vi "(FPGA)_PIDXYZ_laserPID)_COMtemp.vi"() -> ()   [LabVIEW 2018]
doc: "This VI will read single point values from 4 channels of a R Series board at a specified rate."
uses:
  <vilib>/rvi/Emulation/niFpgaGetClockAttributes.vi
  <vilib>/rvi/Emulation/niFpgaSctlEmulationGetInTimedLoop.vi
  <vilib>/rvi/Emulation/niFpgaEmulationReportErrorSimple.vi
  <vilib>/rvi/Emulation/niFpgaProcessEmulError.vi
  <vilib>/rvi/eio/common/nirviEmuTemplateMethod_errors.vi
  <vilib>/rvi/Emulation/niFpgaCriticalErrorInLSC.vi
  <vilib>/rvi/Memory/Memory_Emulation/nirvimemoryFastEmulation.vi
  <vilib>/rvi/Memory/Memory_Emulation/nirvimemoryEmulation.vi
  <vilib>/rvi/Emulation/niFpgaEmulationIsFPGAContextNoSignature.vi
  <vilib>/rvi/DataTransferAndStorage/Container/Common/niFpgaContainerGetUniqueNameForEmu.vi
  <vilib>/rvi/errors/nirviReportUnexpectedCaseInternalError (U32).vi
  <vilib>/rvi/Memory/Memory_Emulation/niFpgaMemoryEmulationCacheClearOnFirstRun.vi
  <vilib>/rvi/Memory/Memory_Emulation/nirvimemoryEmulationManagerCache_MakeExclusive.vi
  <vilib>/rvi/Memory/Memory_Emulation/niFpgaMemoryEmulationValidateCache.vi
  <vilib>/rvi/Memory/Memory_Emulation/nirvimemoryEmulationManagerCache_InsertValue.vi
  <vilib>/Utility/error.llb/Clear Errors.vi
  <vilib>/rvi/Memory/Memory_Emulation/nirvimemoryEmulationManagerCache_ReleaseExclusive.vi
  <vilib>/rvi/Memory/Memory_Emulation/nirvimemoryEmulationManagerCache_GetValue.vi
  <vilib>/rvi/Memory/Memory_Emulation/nirvimemoryEmulationManagerCache_SetValue.vi
  <vilib>/rvi/Emulation/niFpgaSctlEmulationResourceMgr.vi
  <vilib>/eio/EIONode/EIONode.xnode
  <vilib>/rvi/DataTransferAndStorage/Container/XNode/niFpgaContainer.xnode
  <vilib>/rvi/FXPMathLib/FxpInterpret/XNode/nifxpmath_Interpret.xnode
panel:
  in  "Big Number":sgl
  in  "Amplitude_sine_EOM":sgl
  in  "eom sine frequency (periods/tick)":fxp<+,32,0>=0.0002500000409781933
  in  "pz?":bool
  out "pg Z mod":fxp<+/-,24,12>
  in  "pg Z":fxp<+/-,24,12>
  in  "amplitude":i16=8192
  in  "offset":i16=8192
  out "Trigger for COM out":i16 caption="square wave out"
  out "dgz mod":fxp<+/-,24,12>
  in  "activate COMz":bool
  in  "dg Z":fxp<+/-,24,12>
  in  "activate COMy":bool
  out "dgy mod":fxp<+/-,24,12>
  in  "dg Y":fxp<+/-,24,12>
  out "dgx mod":fxp<+/-,24,12>
  in  "activate COMx":bool
  in  "dg X":fxp<+/-,24,12>
  in  "duty cycle (periods)":fxp<+,32,0>=0.5
  in  "frequency (periods/tick)":fxp<+,32,0>=0.00390625
  in  "final filter coeff X before":i32[](array[numeric])=[-955995012, 2025731616, 1001305, -1023351008, 2092954700, 1034533]
  in  "final filter coeff X":i32[](array[numeric])=[-955995012, 2025731616, 1001305, -1023351008, 2092954700, 1034533]
  in  "final filter coeff Y before":i32[](array[numeric])=[-955995012, 2025731616, 1001305, -1023351008, 2092954700, 1034533]
  in  "final filter coeff Y":i32[](array[numeric])=[-955995012, 2025731616, 1001305, -1023351008, 2092954700, 1034533]
  in  "final filter coeff Z":i32[](array[numeric])=[-955995012, 2025731616, 1001305, -1023351008, 2092954700, 1034533]
  in  "final filter coeff Z before":i32[](array[numeric])=[-955995012, 2025731616, 1001305, -1023351008, 2092954700, 1034533]
  in  "LP Coeff Z before":i32[](array[numeric])=[1008310688, 32715568]
  in  "LP Coeff Z":i32[](array[numeric])=[1008310688, 32715568]
  in  "LP Coeff X":i32[](array[numeric])=[1008310688, 32715568]
  in  "LP Coeff X before":i32[](array[numeric])=[1008310688, 32715568]
  in  "LP Coeff Y before":i32[](array[numeric])=[1008310688, 32715568]
  in  "LP Coeff Y":i32[](array[numeric])=[1008310688, 32715568]
  in  "Upper lim Z before":fxp<+/-,16,16>
  in  "Lower lim Z before":fxp<+/-,16,16>
  in  "Upper lim Y before":fxp<+/-,16,16>
  in  "Lower lim Y before":fxp<+/-,16,16>
  in  "Upper lim X before":fxp<+/-,16,16>
  in  "Lower lim X before":fxp<+/-,16,16>
  in  "HP coeff band X before":i32[](array[numeric])=[-850883994, 1909449570, 958518847, -975456236, 2033039520, 1020559395]
  in  "LP Coeff band X before":i32[](array[numeric])=[-955995012, 2025731616, 1001305, -1023351008, 2092954700, 1034533]
  in  "LP Coeff band X":i32[](array[numeric])=[-955995012, 2025731616, 1001305, -1023351008, 2092954700, 1034533]
  in  "HP Coeff band X":i32[](array[numeric])=[-850883994, 1909449570, 958518847, -975456236, 2033039520, 1020559395]
  in  "dg band X before":fxp<+/-,24,12>
  in  "dg band X":fxp<+/-,24,12>
  in  "HP Coeff X before":i32[](array[numeric])=[946630756, 1010186290]
  in  "HP Coeff X":i32[](array[numeric])=[946630756, 1010186290]
  in  "Use X PID before":bool
  out "AI X before chamber plot":i16
  in  "X before Setpoint":i16
  out "tot_fb X plot":i16
  out "fb X before chamber plot":i16
  in  "DC offset X":i16
  in  "pg X before":fxp<+/-,24,12>
  in  "ig X before":fxp<+/-,24,-4>
  in  "dg X before":fxp<+/-,24,12>
  out "fb X plot":i16
  in  "ig X":fxp<+/-,24,-4>
  in  "Lower lim X":fxp<+/-,16,16>
  in  "Upper lim X":fxp<+/-,16,16>
  in  "pg X":fxp<+/-,24,12>
  out "AI X plot":i16
  in  "X Setpoint":i16
  in  "HP coeff band Y before":i32[](array[numeric])=[-850883994, 1909449570, 958518847, -975456236, 2033039520, 1020559395]
  in  "LP Coeff band Y before":i32[](array[numeric])=[-955995012, 2025731616, 1001305, -1023351008, 2092954700, 1034533]
  in  "LP Coeff band Y":i32[](array[numeric])=[-955995012, 2025731616, 1001305, -1023351008, 2092954700, 1034533]
  in  "HP Coeff band Y":i32[](array[numeric])=[-850883994, 1909449570, 958518847, -975456236, 2033039520, 1020559395]
  in  "dg band Y before":fxp<+/-,24,12>
  in  "dg band Y":fxp<+/-,24,12>
  in  "HP Coeff Y before":i32[](array[numeric])=[946630756, 1010186290]
  in  "HP Coeff Y":i32[](array[numeric])=[946630756, 1010186290]
  in  "Use Y PID before":bool
  out "AI Y before chamber plot":i16
  in  "Y before Setpoint":i16
  out "tot_fb Y plot":i16
  out "fb Y before chamber plot":i16
  in  "DC offset Y":i16
  in  "pg Y before":fxp<+/-,24,12>
  in  "ig Y before":fxp<+/-,24,-4>
  in  "dg Y before":fxp<+/-,24,12>
  out "fb Y plot":i16
  in  "ig Y":fxp<+/-,24,-4>
  in  "Lower lim Y":fxp<+/-,16,16>
  in  "Upper lim Y":fxp<+/-,16,16>
  in  "pg Y":fxp<+/-,24,12>
  out "AI Y plot":i16
  in  "Y Setpoint":i16
  in  "EOM_offset":i16
  in  "EOM_seed":u32=4294967295 caption="seed"
  in  "EOM reset":bool caption="reset"
  in  "EOM_threshold":i16
  in  "EOM_amplitude":i16
  in  "HP coeff band Z before":i32[](array[numeric])=[-850883994, 1909449570, 958518847, -975456236, 2033039520, 1020559395]
  in  "LP Coeff band Z before":i32[](array[numeric])=[-955995012, 2025731616, 1001305, -1023351008, 2092954700, 1034533]
  in  "LP Coeff band Z":i32[](array[numeric])=[-955995012, 2025731616, 1001305, -1023351008, 2092954700, 1034533]
  in  "HP Coeff band Z":i32[](array[numeric])=[-850883994, 1909449570, 958518847, -975456236, 2033039520, 1020559395]
  in  "dg band Z before":fxp<+/-,24,12>
  in  "dg band Z":fxp<+/-,24,12>
  in  "data_buffer3":i16
  in  "Arb gain (ch2)":fxp<+/-,24,12>=0.5 caption="RMS"
  in  "HP Coeff Z before":i32[](array[numeric])=[946630756, 1010186290]
  in  "HP Coeff Z":i32[](array[numeric])=[946630756, 1010186290]
  in  "Use Z PID before":bool
  out "AI Z before chamber plot":i16
  in  "Z before Setpoint":i16
  out "tot_fb Z plot":i16
  out "fb Z before chamber plot":i16
  in  "DC offset Z":i16
  in  "pg Z before":fxp<+/-,24,12>
  in  "ig Z before":fxp<+/-,24,-4>
  in  "dg Z before":fxp<+/-,24,12>
  out "fb Z plot":i16
  in  "ig Z":fxp<+/-,24,-4>
  out "written_address":u32
  in  "ready_to_write":bool
  in  "Arb steps per cycle":u16
  in  "data_buffer2":i16
  in  "data_buffer_1":i16
  in  "write_address":u16
  in  "Arb gain (ch1)":fxp<+/-,24,12>=0.5 caption="RMS"
  in  "Arb gain (ch0)":fxp<+/-,24,12>=0.5 caption="RMS"
  in  "Lower lim Z":fxp<+/-,16,16>
  in  "Upper lim Z":fxp<+/-,16,16>
  out "AI Z plot":i16
  in  "Z Setpoint":i16
  in  "Count(uSec)":u32
  out "FPGA Error Out":errorcluster
  in  "Stop":bool
  # "test"
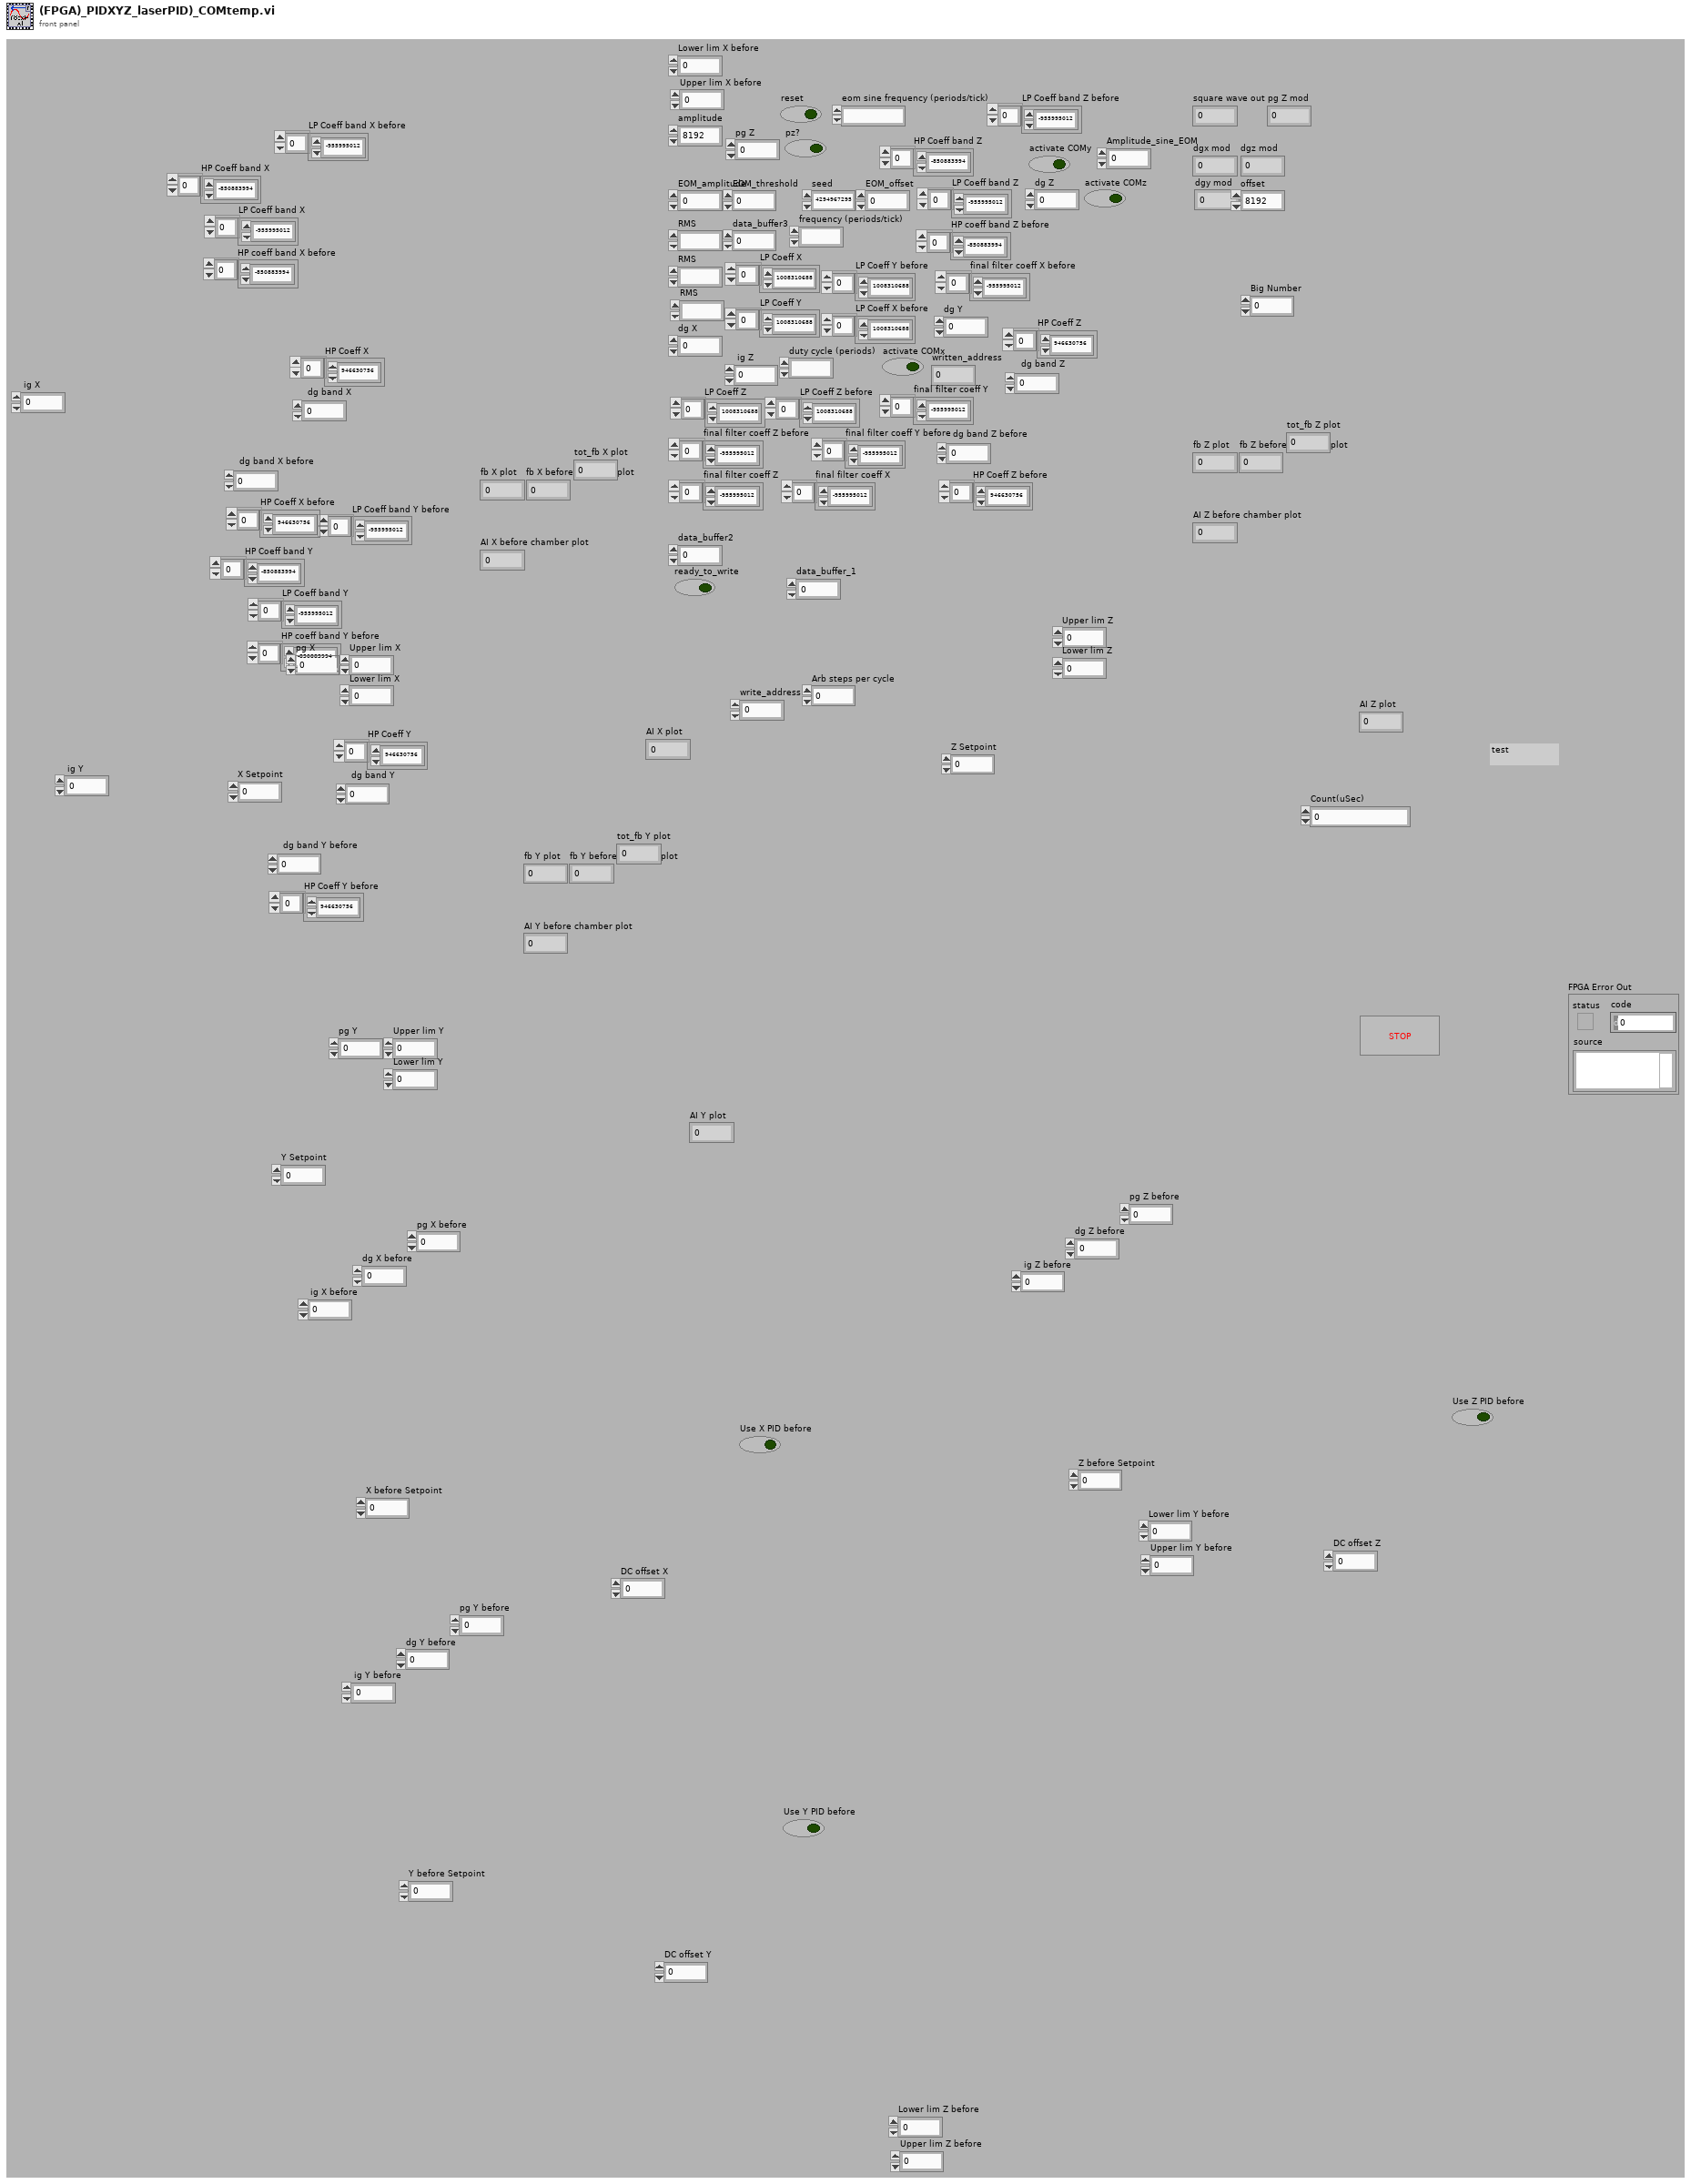
[diagram p1: front panel]
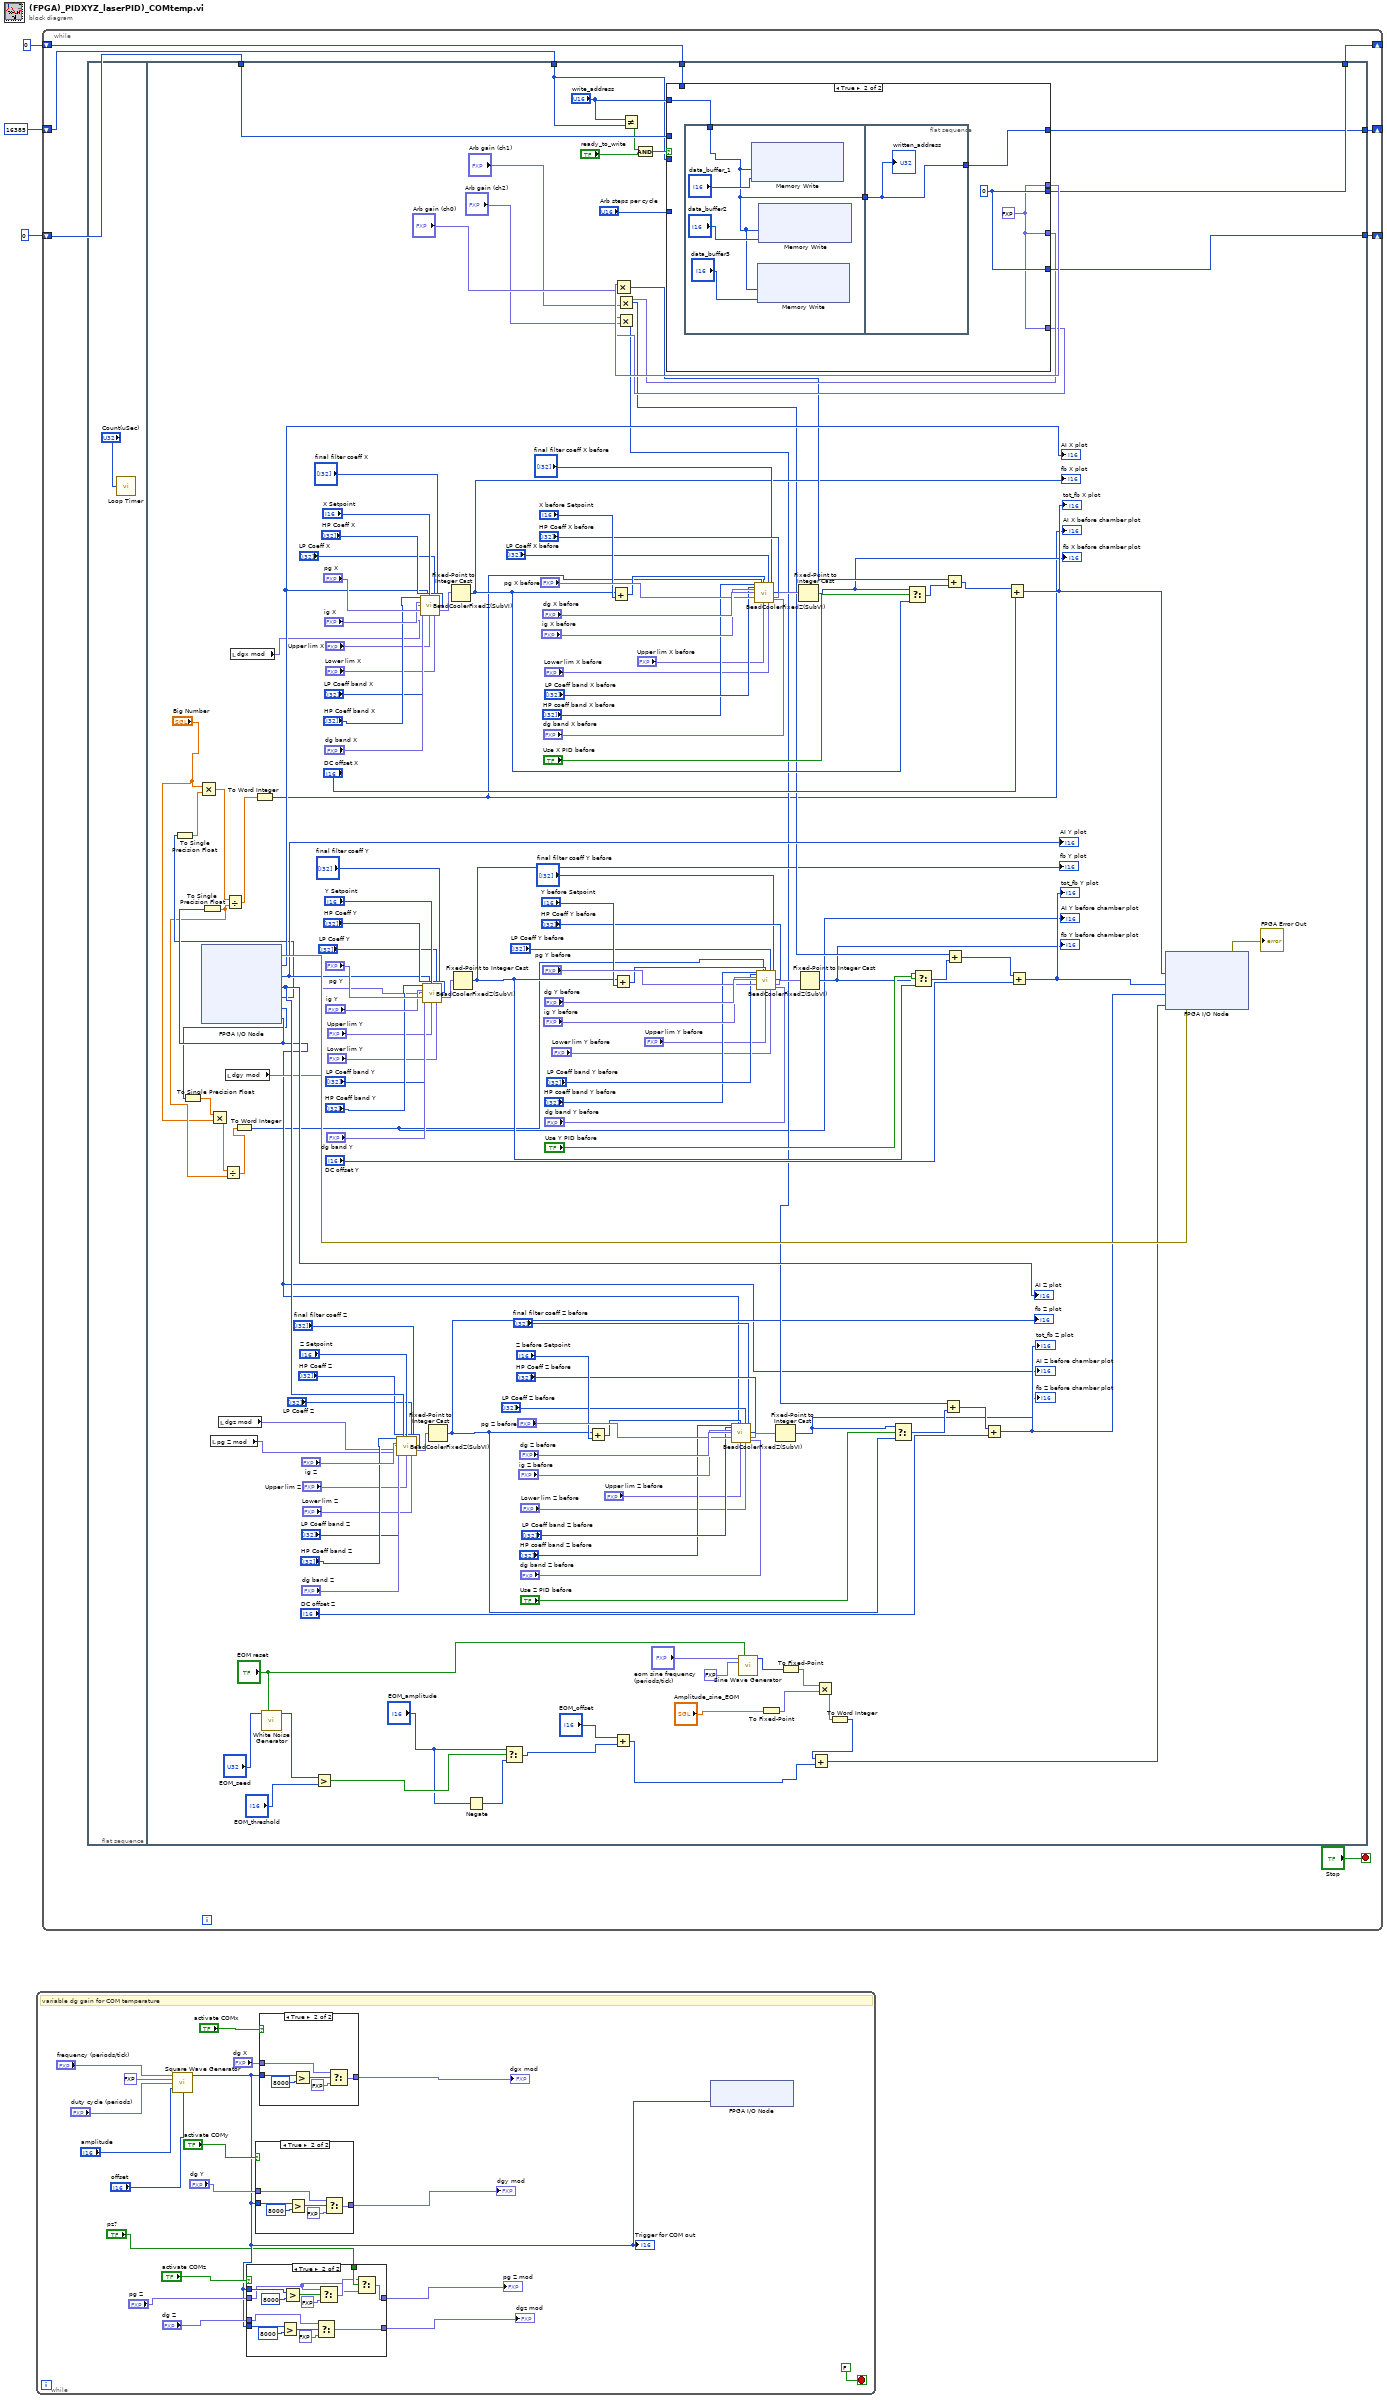
[diagram p0: block diagram]
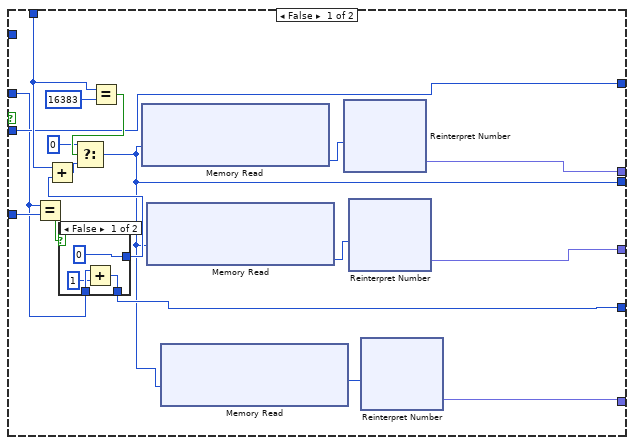
[diagram p5: hidden frame]
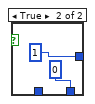
[diagram p6: hidden frame]
diagram:
  n1 = while {
    stop <- FALSE stop-if-true
    # "variable dg gain for COM temperature"
    n2 = call "Square Wave Generator"("frequency (periods/tick)"="frequency (periods/tick)", "phase offset (periods)"=fxp<+,32,0> 0.0, "duty cycle (periods)"="duty cycle (periods)", "amplitude"="amplitude", "offset"="offset") -> ("square wave out"=w5:i16)  [unwired: 10 in]
    "Trigger for COM out" <- w5
    n3 = case shown="True" "activate COMz" {
      tunnel: [w24 w35] -> w8
      tunnel: w5 -> [_ w38]
      tunnel: "dg Z" -> [w24 w33]
      tunnel: "pg Z" -> [w23 w25]
      tunnel: [w23 w26] -> w6
      tunnel: w5 -> [_ w29]
      tunnel: "pz?" -> [_ w28]
      frame False {
      }
      frame True {
        n4 = Greater?(x=w38, y=i16 8000) -> (0:w36:bool)
        n5 = Greater?(x=w29, y=i16 8000) -> (0:w31:bool)
        n6 = Select(t=w33, s=w36, f=fxp<+/-,24,12> 0.0 ("y")) -> (s? t:f=w35:fxp<+/-,24,12>)
        n7 = Select(t=w25, s=w31, f=fxp<+/-,24,12> 0.0 ("y")) -> (s? t:f=w27:fxp<+/-,24,12>)
        n8 = Select(t=w27, s=w28, f=w25) -> (s? t:f=w26:fxp<+/-,24,12>)
      }
    }
    "dgz mod" <- w8
    "pg Z mod" <- w6
    n9 = case shown="True" "activate COMy" {
      tunnel: "dg Y" -> [w39 w41]
      tunnel: [w39 w42] -> w12
      tunnel: w5 -> [_ w45]
      frame False {
      }
      frame True {
        n10 = Greater?(x=w45, y=i16 8000) -> (0:w43:bool)
        n11 = Select(t=w41, s=w43, f=fxp<+/-,24,12> 0.0 ("y")) -> (s? t:f=w42:fxp<+/-,24,12>)
      }
    }
    "dgy mod" <- w12
    n12 = case shown="True" "activate COMx" {
      tunnel: "dg X" -> [w46 w48]
      tunnel: [w46 w49] -> w14
      tunnel: w5 -> [_ w52]
      frame False {
      }
      frame True {
        n13 = Greater?(x=w52, y=i16 8000) -> (0:w50:bool)
        n14 = Select(t=w48, s=w50, f=fxp<+/-,24,12> 0.0 ("y")) -> (s? t:f=w49:fxp<+/-,24,12>)
      }
    }
    "dgx mod" <- w14
    n15 = xnode "FPGA I/O Node"("Connector0/AO7"=w5) -> ()  [unwired: 2 in, 2 out]
  }
  n16 = while {
    shift-right: [w58] -> _
    shift-left: u16 0 ("t") -> [w57]
    shift-right: [w56] -> _
    shift-left: u16 0 ("t") -> [w53]
    shift-right: [w55] -> _
    shift-left: u32 16385 ("write_address") -> [w54]
    stop <- "Stop" stop-if-true
    n17 = flat-sequence {
      tunnel: [w214] -> w58
      tunnel: w57 -> [w213]
      tunnel: [w211] -> w56
      tunnel: w53 -> [w210]
      tunnel: [w209] -> w55
      tunnel: w54 -> [w202]
      frame #0 {
        n18 = call "Loop Timer"("Count(uSec)"="Count(uSec)") -> ()  [unwired: 1 out]
      }
      frame #1 {
        n19 = xnode "FPGA I/O Node"() -> ("error out"=w219:errorcluster, "Connector0/AI0"=w123:i16, "Connector0/AI1"=w147:i16, "Connector0/AI2"=w200:i16, "Connector0/AI3"=w68:i16, "Connector0/AI4"=w67:i16, "Connector0/AI5"=w72:i16)  [unwired: 7 in, 6 out]
        "AI Z plot" <- w200
        "AI Z before chamber plot" <- w72
        "AI Y plot" <- w147
        "AI X plot" <- w123
        n20 = To Single Precision Float(number=w68) -> (single precision float=w71:sgl)
        n21 = To Single Precision Float(number=w67) -> (single precision float=w66:sgl)
        n22 = Multiply(x="Big Number", y=w71) -> (x*y=w70:sgl)
        n23 = To Single Precision Float(number=w72) -> (single precision float=w64:sgl)
        n24 = Multiply(x=w66, y="Big Number") -> (x*y=w65:sgl)
        n25 = local read "pg Z mod"() -> (w85:fxp<+/-,24,12>)
        n26 = local read "dgz mod"() -> (w86:fxp<+/-,24,12>)
        n27 = Divide(x=w65, y=w64) -> (x/y=w63:sgl)
        n28 = Divide(x=w70, y=w64) -> (x/y=w69:sgl)
        n29 = local read "dgy mod"() -> (w87:fxp<+/-,24,12>)
        n30 = local read "dgx mod"() -> (w88:fxp<+/-,24,12>)
        n31 = To Word Integer(number=w63) -> (16bit integer=w62:i16)
        "AI Y before chamber plot" <- w62
        n32 = To Word Integer(number=w69) -> (16bit integer=w73:i16)
        "AI X before chamber plot" <- w73
        n33 = call "White Noise Generator"("seed"="EOM_seed", "reset"="EOM reset") -> ("white noise out"=w179:i16)  [unwired: 13 in]
        n34 = Greater?(x=w179, y="EOM_threshold") -> (0:w177:bool)
        n35 = call "BeadCoolerFixedZ(SubVI).vi"("hp coeff band"="HP Coeff band Z", "lp coeff band"="LP Coeff band Z", "ig"="ig Z", "dg"=w86, "pg"=w85, "dg band"="dg band Z", "AI0"=w200, "Dc Pos"="Z Setpoint", "Upper lim"="Upper lim Z", "lp coeff"="LP Coeff Z", "Lower lim"="Lower lim Z", "final filter coeff"="final filter coeff Z", "hp coeff"="HP Coeff Z") -> ("Output"=w189:fxp<+/-,16,16>)  [unwired: 14 in]
        n36 = call "BeadCoolerFixedZ(SubVI).vi"("hp coeff band"="HP Coeff band X", "lp coeff band"="LP Coeff band X", "ig"="ig X", "dg"=w88, "pg"="pg X", "dg band"="dg band X", "AI0"=w123, "Dc Pos"="X Setpoint", "Upper lim"="Upper lim X", "lp coeff"="LP Coeff X", "Lower lim"="Lower lim X", "final filter coeff"="final filter coeff X", "hp coeff"="HP Coeff X") -> ("Output"=w133:fxp<+/-,16,16>)  [unwired: 14 in]
        n37 = call "BeadCoolerFixedZ(SubVI).vi"("hp coeff band"="HP Coeff band Y", "lp coeff band"="LP Coeff band Y", "ig"="ig Y", "dg"=w87, "pg"="pg Y", "dg band"="dg band Y", "AI0"=w147, "Dc Pos"="Y Setpoint", "Upper lim"="Upper lim Y", "lp coeff"="LP Coeff Y", "Lower lim"="Lower lim Y", "final filter coeff"="final filter coeff Y", "hp coeff"="HP Coeff Y") -> ("Output"=w157:fxp<+/-,16,16>)  [unwired: 14 in]
        n38 = Fixed-Point to Integer Cast(1:w189) -> (0:w98:i16)
        "fb Z plot" <- w98
        n39 = Fixed-Point to Integer Cast(1:w133) -> (0:w102:i16)
        "fb X plot" <- w102
        n40 = Fixed-Point to Integer Cast(1:w157) -> (0:w100:i16)
        "fb Y plot" <- w100
        n41 = Negate(x="EOM_amplitude") -> (-x=w175:i16)
        n42 = Select(t="EOM_amplitude", s=w177, f=w175) -> (s? t:f=w173:i16)
        n43 = Add(x=w98, y="Z before Setpoint") -> (x+y=w188:i16)
        n44 = Add(x=w102, y="X before Setpoint") -> (x+y=w132:i16)
        n45 = Add(x=w100, y="Y before Setpoint") -> (x+y=w156:i16)
        n46 = Add(x="EOM_offset", y=w173) -> (x+y=w76:i16)
        n47 = Not Equal?(x="write_address", y=w202) -> (x != y?=w206:bool)
        n48 = And(x=w206, y="ready_to_write") -> (x .and. y?=w207:bool)
        n49 = case shown="True" w207 {
          tunnel: [w236 w244] -> w216
          tunnel: [w221 w248] -> w214
          tunnel: w213 -> [w229 _]
          tunnel: [w230 w244] -> w204
          tunnel: "Arb steps per cycle" -> [w228 _]
          tunnel: [w223 w248] -> w211
          tunnel: w210 -> [w224 _]
          tunnel: [w227 w246] -> w209
          tunnel: w202 -> [w227 _]
          tunnel: "write_address" -> [_ w245]
          tunnel: [w220 w244] -> w186
          frame False {
            n50 = Equal?(x=w224, y=w228) -> (x = y?=w226:bool)
            n51 = case shown="False" w226 {
              tunnel: [u16 0 ("y") u16 1 ("y")] -> w225
              tunnel: w224 -> [w240 _]
              tunnel: [w238 u16 0] -> w223
              frame False {
                n52 = Add(x=w240, y=u16 1) -> (x+y=w238:u16)
              }
              frame True {
              }
            }
            n53 = Add(x=w229, y=w225) -> (x+y=w232:u16)
            n54 = Equal?(x=w229, y=u16 16383) -> (x = y?=w234:bool)
            n55 = Select(t=u16 0, s=w234, f=w232) -> (s? t:f=w221:u16)
            n56 = xnode ("Memory Read")("Address"=w221) -> ("Data"=w237:i16)  [unwired: 1 in, 1 out]
            n57 = xnode ("Memory Read")("Address"=w221) -> ("Data"=w231:i16)  [unwired: 1 in, 1 out]
            n58 = xnode ("Memory Read")("Address"=w221) -> ("Data"=w222:i16)  [unwired: 1 in, 1 out]
            n59 = xnode "Reinterpret Number"("x"=w237) -> ("y"=w236:fxp<+/-,16,16>)
            n60 = xnode "Reinterpret Number"("x"=w231) -> ("y"=w230:fxp<+/-,16,16>)
            n61 = xnode "Reinterpret Number"("x"=w222) -> ("y"=w220:fxp<+/-,16,16>)
          }
          frame True {
            w248 = u16 0
            w244 = fxp<+/-,16,16> 0.0 ("y")
            n62 = flat-sequence {
              tunnel: [w250] -> w247
              tunnel: w245 -> [w250]
              tunnel: w247 -> [w253]
              tunnel: [w253] -> w246
              frame #0 {
                n63 = xnode ("Memory Write")("Address"=w250, "Data"="data_buffer_1") -> ()  [unwired: 1 in, 1 out]
                n64 = xnode ("Memory Write")("Address"=w250, "Data"="data_buffer3") -> ()  [unwired: 1 in, 1 out]
                n65 = xnode ("Memory Write")("Address"=w250, "Data"="data_buffer2") -> ()  [unwired: 1 in, 1 out]
              }
              frame #1 {
                "written_address" <- w253
              }
            }
          }
        }
        n66 = Multiply(x=w216, y="Arb gain (ch0)") -> (x*y=w103:i16)
        n67 = Multiply(x=w204, y="Arb gain (ch1)") -> (x*y=w101:i16)
        n68 = Multiply(x=w186, y="Arb gain (ch2)") -> (x*y=w99:i16)
        n69 = call "BeadCoolerFixedZ(SubVI).vi"("hp coeff band"="HP coeff band Z before", "lp coeff band"="LP Coeff band Z before", "ig"="ig Z before", "dg"="dg Z before", "pg"="pg Z before", "dg band"="dg band Z before", "AI0"=w72, "Dc Pos"=w188, "Upper lim"="Upper lim Z before", "lp coeff"="LP Coeff Z before", "Lower lim"="Lower lim Z before", "final filter coeff"="final filter coeff Z before", "hp coeff"="HP Coeff Z before") -> ("Output"=w196:fxp<+/-,16,16>)  [unwired: 14 in]
        n70 = call "Sine Wave Generator"("frequency (periods/tick)"="eom sine frequency (periods/tick)", "reset"="EOM reset", "phase offset (periods)"=fxp<+,32,0> 0.0) -> ("sine out"=w82:i16)  [unwired: 12 in]
        n71 = call "BeadCoolerFixedZ(SubVI).vi"("hp coeff band"="HP coeff band X before", "lp coeff band"="LP Coeff band X before", "ig"="ig X before", "dg"="dg X before", "pg"="pg X before", "dg band"="dg band X before", "AI0"=w73, "Dc Pos"=w132, "Upper lim"="Upper lim X before", "lp coeff"="LP Coeff X before", "Lower lim"="Lower lim X before", "final filter coeff"="final filter coeff X before", "hp coeff"="HP Coeff X before") -> ("Output"=w139:fxp<+/-,16,16>)  [unwired: 14 in]
        n72 = call "BeadCoolerFixedZ(SubVI).vi"("hp coeff band"="HP coeff band Y before", "lp coeff band"="LP Coeff band Y before", "ig"="ig Y before", "dg"="dg Y before", "pg"="pg Y before", "dg band"="dg band Y before", "AI0"=w62, "Dc Pos"=w156, "Upper lim"="Upper lim Y before", "lp coeff"="LP Coeff Y before", "Lower lim"="Lower lim Y before", "final filter coeff"="final filter coeff Y before", "hp coeff"="HP Coeff Y before") -> ("Output"=w163:fxp<+/-,16,16>)  [unwired: 14 in]
        n73 = To Fixed-Point(number="Amplitude_sine_EOM") -> (fixed-point=w80:fxp<+/-,32,16>)  [unwired: 1 in]
        n74 = Fixed-Point to Integer Cast(1:w196) -> (0:w89:i16)
        "fb Z before chamber plot" <- w89
        n75 = To Fixed-Point(number=w82) -> (fixed-point=w81:fxp<+/-,16,16>)  [unwired: 1 in]
        n76 = Fixed-Point to Integer Cast(1:w139) -> (0:w95:i16)
        "fb X before chamber plot" <- w95
        n77 = Fixed-Point to Integer Cast(1:w163) -> (0:w92:i16)
        "fb Y before chamber plot" <- w92
        n78 = Multiply(x=w81, y=w80) -> (x*y=w79:fxp<+/-,48,32>)
        n79 = To Word Integer(number=w79) -> (16bit integer=w77:i16)
        n80 = Add(x=w77, y=w76) -> (x+y=w75:i16)
        n81 = Select(t=w89, s="Use Z PID before", f=w98) -> (s? t:f=w91:i16)
        n82 = Select(t=w95, s="Use X PID before", f=w102) -> (s? t:f=w97:i16)
        n83 = Select(t=w92, s="Use Y PID before", f=w100) -> (s? t:f=w94:i16)
        n84 = Add(x=w99, y=w91) -> (x+y=w90:i16)
        n85 = Add(x=w103, y=w97) -> (x+y=w96:i16)
        n86 = Add(x=w101, y=w94) -> (x+y=w93:i16)
        n87 = Add(x=w90, y="DC offset Z") -> (x+y=w192:i16)
        "tot_fb Z plot" <- w192
        n88 = Add(x=w96, y="DC offset X") -> (x+y=w122:i16)
        "tot_fb X plot" <- w122
        n89 = Add(x=w93, y="DC offset Y") -> (x+y=w146:i16)
        "tot_fb Y plot" <- w146
        n90 = xnode "FPGA I/O Node"("error in"=w219, "Connector0/AO0"=w122, "Connector0/AO1"=w146, "Connector0/AO2"=w192, "Connector0/AO3"=w75) -> ("error out"=→"FPGA Error Out":errorcluster)  [unwired: 4 in, 4 out]
      }
    }
  }
